vi "stream.vi"(8 "error in":errorcluster, 9 "Data":T1(array[cluster]), 10 "Data Source RID":string, 11 "Nominal Client in":refnum<class "Nominal Client.lvclass">) -> (0 "error out":errorcluster, 3 "Nominal Client out":refnum<class "Nominal Client.lvclass">, 4 "Response body":string)   [LabVIEW 2024, in "nominal labview client.lvlib"]
uses:
  nominal labview client.lvlib
  <vilib>/Nominal/Nominal IO Client/Nominal Client/Nominal Client.lvclass
  b76046d4-2b9b-4960-9c02-6271b4e5d39a.vi
  18f79811-cb16-469d-8a6d-9a6241d3ffe4.vi
  18f79811-cb16-469d-8a6d-9a6241d3ffe4.vi/cdde0a50-1f2d-45b6-8c5c-67b334d1f5bb.vi
  18f79811-cb16-469d-8a6d-9a6241d3ffe4.vi/2aaf4cd1-b7d0-4e89-be55-e948b2020e34.vi
  <vilib>/LabVIEW Open Source Project/Epoch Date & Time/epoch.UNIX/Epoch.UNIX.lvclass
  <vilib>/LabVIEW Open Source Project/Epoch Date & Time/Get Epoch Time.vi
  <vilib>/JDP Science/JSONtext/Variant to JSON Text.vi
  <vilib>/JDP Science/JSONtext/Array of Variants to JSON Object.vi
  <vilib>/JDP Science/JSONtext/Set Item.vi
  <vilib>/Nominal/Nominal IO Client/Nominal Client/http.post.vi
  <vilib>/JDP Science/JSONtext/LVClass Serializer/JSONtext LVClass Serializer.lvclass
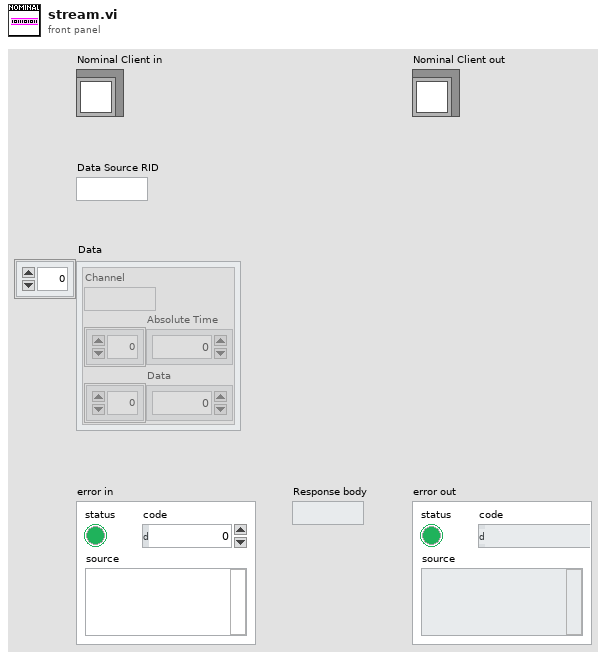
[diagram p1: front panel]
types:
  T1 = cluster{"Channel":string, "Absolute Time":dbl[], "Data":dbl[]}[]
  T2 = cluster{"UNIX Timestamp":cluster{"Seconds":i64, "Nanoseconds":i64}, "Absolute Time":dbl}
  T3 = cluster{"Channel":string, cluster{"UNIX Timestamp":cluster{"Seconds":i64, "Nanoseconds":i64}, "Absolute Time":dbl}[]}
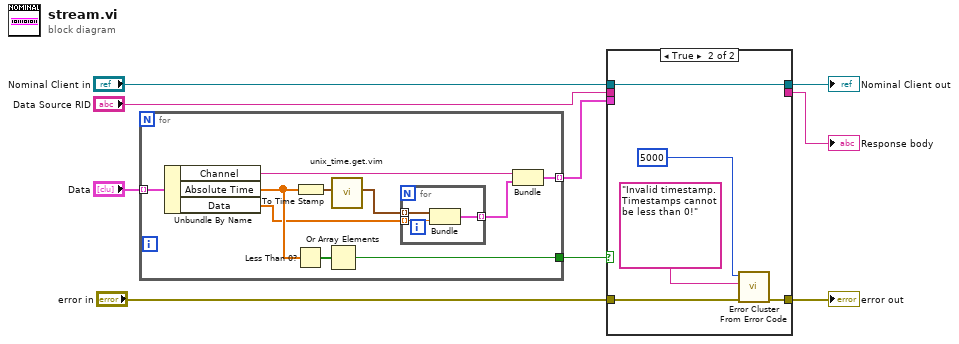
[diagram p0: block diagram]
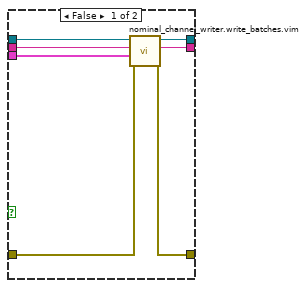
[diagram p2: hidden frame]
diagram:
  n1 = for {
    tunnel: [w19] -> w8 mode=indexing
    tunnel: "Data" -> [w18] mode=indexing
    tunnel: [w10] -> w1
    n2 = Unbundle By Name(w18) -> ("Channel"=w14:string, "Absolute Time"=w13:dbl[], "Data"=w11:dbl[])
    n3 = Less Than 0?(x=w13) -> (x < 0?=w12:bool[])
    n4 = To Time Stamp(1:w13) -> (0:w17:timestamp[])
    n5 = Or Array Elements(Boolean array=w12) -> (logical OR=w10:bool)
    n6 = call "unix_time.get.vim"("Time Stamp (empty: now) [single or array]"=w17) -> ("UNIX Timestamp"=w16:cluster{"Seconds":i64, "Nanoseconds":i64}[])  [unwired: 10 in]
    n7 = for {
      tunnel: w11 -> [w20] mode=indexing
      tunnel: w16 -> [w21] mode=indexing
      tunnel: [w22] -> w15 mode=indexing
      n8 = Bundle("UNIX Timestamp"=w21, "Absolute Time"=w20) -> (w22:T2)  [unwired: 1 in]
    }
    n9 = Bundle("Channel"=w14, w15) -> (w19:T3)  [unwired: 1 in]
  }
  n10 = case shown="True" w1 {
    tunnel: "Data Source RID" -> [w29 _]
    tunnel: w8 -> [w28 _]
    tunnel: "Nominal Client in" -> [w27 w34]
    tunnel: [w26 w34] -> w5
    tunnel: [w25 w30] -> w4
    tunnel: "error in" -> [w24 w31]
    tunnel: [w23 _] -> w2
    frame False {
      n11 = call "nominal_channel_writer.write_batches.vim"("error in"=w24, "batches"=w28, "Data Source RID"=w29, "Nominal Client in"=w27) -> ("error out"=w25:errorcluster, "Response body"=w23:string, "Nominal Client out"=w26:refnum<class "Nominal Client.lvclass">)  [unwired: 5 in]
    }
    frame True {
      n12 = call <vilib>:"Error Cluster From Error Code.vi"("error in (no error)"=w31, "error message (\"\")"="Invalid timestamp. Timestamps cannot be less than 0!" ("error message (\"\")"), "error code (0)"=5000) -> ("error out"=w30:errorcluster)  [unwired: 6 in]
    }
  }
  "Nominal Client out" <- w5
  "error out" <- w4
  "Response body" <- w2
